vi "Run.vi"(8 "error in (no error)":errorcluster caption="entrée d'erreur (pas d'erreur)", 9 "labels_pred":string[][](array[string]), 10 "labels_true":string[][](array[string]), 11 "Homogeneity_C_V_M.lvclass":refnum<class "Homogeneity_C_V_M.lvclass">) -> (0 "error out":errorcluster caption="sortie d'erreur", 2 "String Data":string, 3 "Homogeneity_C_V_M.lvclass":refnum<class "Homogeneity_C_V_M.lvclass">)   [LabVIEW 2020, in "Homogeneity_C_V_M.lvclass"]
doc: "Returns : \n\n- homogeneity : float\nscore between 0.0 and 1.0. 1.0 stands for perfectly homogeneous labeling\n\n- completeness : float\nscore between 0.0 and 1.0. 1.0 stands for perfectly complete labeling\n\n- v_measure : float\nharmonic mean of the first two"
uses:
  Homogeneity_C_V_M.lvclass
  Homogeneity_C_V_M.lvclass/Homogeneity_C_V_M.ctl
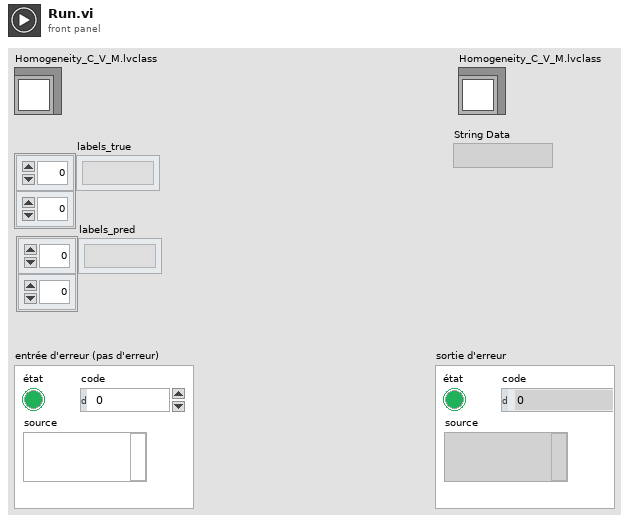
[diagram p1: front panel]
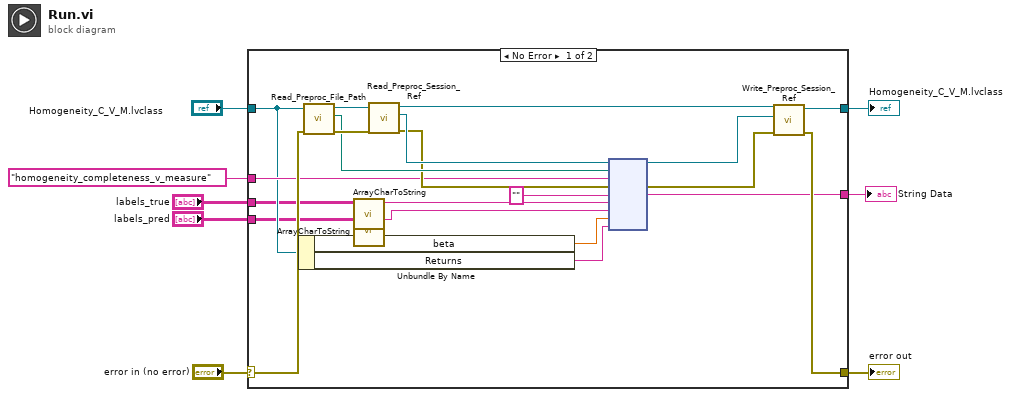
[diagram p0: block diagram]
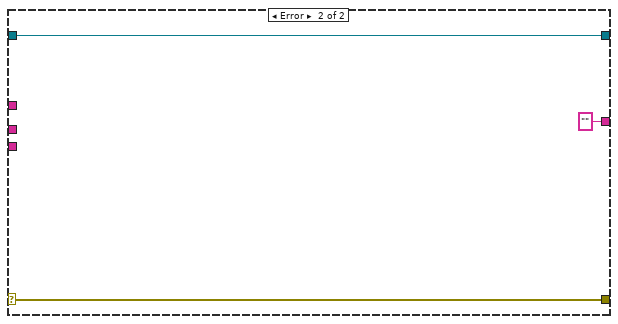
[diagram p2: hidden frame]
diagram:
  n1 = case shown="No Error" "error in (no error)" {
    selector: "error in (no error)" -> [w18 w32]
    tunnel: [w19 w32] -> w7
    tunnel: [w20 w31] -> w5
    tunnel: "Homogeneity_C_V_M.lvclass" -> [w15 w31]
    tunnel: "homogeneity_completeness_v_measure" -> [w17 _]
    tunnel: [w16 ""] -> w4
    tunnel: "labels_true" -> [w12 _]
    tunnel: "labels_pred" -> [w11 _]
    frame No Error {
      n2 = Unbundle By Name(w15) -> ("beta"=w14:dbl, "Returns"=w13:string)
      n3 = call-dynamic "Read_Preproc_File_Path.vi"("error in (no error)"=w18, "Python in"=w15) -> ("error out"=w28:errorcluster, "File_Path"=w27:path, "Python out"=w29:refnum<class "Homogeneity_C_V_M.lvclass">)  [unwired: 7 in]
      n4 = call "ArrayCharToString.vi"("TAB"=w12) -> ("Instruction"=w10:string)  [unwired: 10 in]
      n5 = call "ArrayCharToString.vi"("TAB"=w11) -> ("Instruction"=w9:string)  [unwired: 10 in]
      n6 = call-dynamic "Read_Preproc_Session_Ref.vi"("error in (no error)"=w28, "Python in"=w29) -> ("error out"=w25:errorcluster, "Session_ref"=w26:refnum<k35>, "Python out"=w24:refnum<class "Homogeneity_C_V_M.lvclass">)  [unwired: 7 in]
      n7 = node(w26, w27, w17, w25, "", w10, w9, w14, w13) -> (w22:refnum<k35>, w23:errorcluster, w16:string)  [unwired: 4 in, 2 out]
      n8 = call-dynamic "Write_Preproc_Session_Ref.vi"("error in (no error)"=w23, "Session_ref"=w22, "Python in"=w24) -> ("error out"=w19:errorcluster, "Python out"=w20:refnum<class "Homogeneity_C_V_M.lvclass">)  [unwired: 7 in]
    }
    frame Error {
    }
  }
  "error out" <- w7
  "Homogeneity_C_V_M.lvclass" <- w5
  "String Data" <- w4
